vi "Add Waveform Sections.vi"(8 "error in":errorcluster, 10 "Source Waveform refs in":T1[](array[typedef]) format="%.0x", 11 "CustomDevice Ref":T1 format="%.0x") -> (0 "error out":errorcluster, 1 "Waveform Result Section refs":T1[](array[typedef]) format="%.0x", 2 "Source Waveform refs out":T1[](array[typedef]) format="%.0x", 3 "CustomDevice Ref":T1 format="%.0x")   [LabVIEW 2015, in "Waveform-Processing-Custom-Device System Explorer.lvlib"]
uses:
  Waveform-Processing-Custom-Device System Explorer.lvlib
  <vilib>/NI VeriStand/Custom Device API/Custom Device API.lvlib
  Shared/Constants.vi
  Shared/Waveform-Processing-Custom-Device Shared.lvlib
  <vilib>/NI Veristand/Custom Device API/Set Item Property (Dependent Node Pointer).vi
  NationalInstruments.VeriStand.SystemStorage
  <vilib>/NI Veristand/Custom Device API/Set Item Property (Double).vi
  <vilib>/NI Veristand/Custom Device API/Custom Device Item Ref.ctl
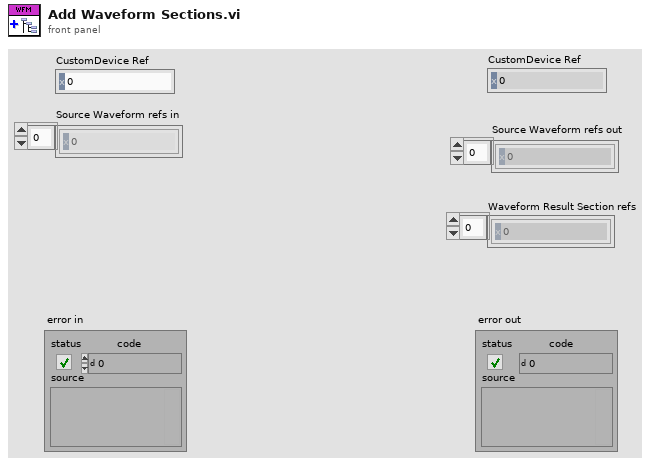
[diagram p1: front panel]
types:
  T1 = typedef "Custom Device API.lvlib/Custom Device Item Ref.ctl" = u64
  T2 = typedef "Custom Device API.lvlib/Custom Device Pointer.ctl" = refnum<k24>
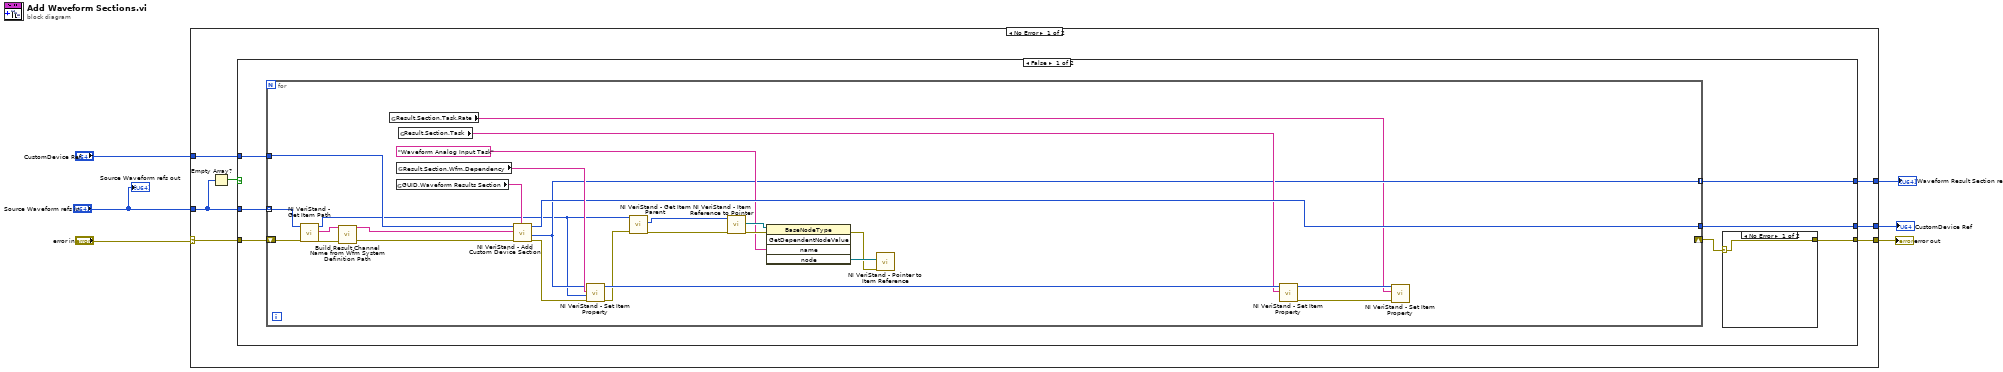
[diagram p0: block diagram]
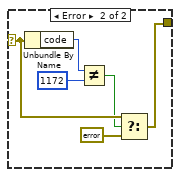
[diagram p2: hidden frame]
diagram:
  n1 = case shown="No Error" "error in" {
    selector: "error in" -> [w12 w57]
    tunnel: [w11 w57] -> w5
    tunnel: "CustomDevice Ref" -> [w13 w56]
    tunnel: [w10 w56] -> w3
    tunnel: [w8 _] -> w2
    tunnel: "Source Waveform refs in" -> [w7 _]
    frame No Error {
      n2 = Empty Array?(array=w7) -> (empty?=w9:bool)
      n3 = case shown="False" w9 {
        tunnel: w13 -> [w20 w55]
        tunnel: w12 -> [w19 w54]
        tunnel: [w16 w54] -> w11
        tunnel: [w18 w55] -> w10
        tunnel: [w15 _] -> w8
        tunnel: w7 -> [w14 _]
        frame False {
          n4 = for {
            tunnel: w20 -> [w53]
            tunnel: [w49] -> w18
            shift-right: [_] -> w17
            shift-left: w19 -> [w37]
            tunnel: [w38] -> w15 mode=indexing
            tunnel: w14 -> [w36] mode=indexing
            n5 = call <vilib>:"NI VeriStand - Get Item Path.vi"("error in (no error)"=w37, "Item Ref in"=w36) -> ("error out"=w34:errorcluster, "Path"=w33:string, "Item Ref out"=w35:T1)  [unwired: 6 in, 1 out]
            n6 = call "Build Result Channel Name from Wfm System Definition Path.vi"("error in (no error)"=w34, "Channel Path"=w33) -> ("error out"=w31:errorcluster, "delimited string"=w32:string)  [unwired: 8 in]
            n7 = global read "Constants.vi" "Result.Section.Task.Rate"() -> (w29:string)
            n8 = global read "Constants.vi" "GUID.Waveform Results Section"() -> (w52:string)
            n9 = global read "Constants.vi" "Result.Section.Wfm.Dependency"() -> (w51:string)
            n10 = global read "Constants.vi" "Result.Section.Task"() -> (w47:string)
            n11 = call <vilib>:"NI VeriStand - Add Custom Device Section.vi"("GUID (Default Section)"=w52, "error in (no error)"=w31, "Section Name"=w32, "Parent Ref in"=w53) -> ("error out"=w50:errorcluster, "Section Ptr"=w38:T1, "Parent Ref out"=w49:T1)  [unwired: 4 in, 1 out]
            n12 = call-poly <vilib>:"NI VeriStand - Set Item Property.vi"("error in (no error)"=w50, "Dependent Node Ref"=w35, "Property Name"=w51, "Item Ref in"=w38) -> ("error out"=w46:errorcluster, "Item Ref out"=w48:T1)  [unwired: 5 in, 1 out]
            n13 = call <vilib>:"NI VeriStand - Get Item Parent.vi"("error in (no error)"=w46, "Item Ref in"=w35) -> ("error out"=w45:errorcluster, "Parent Ref"=w44:T1)  [unwired: 6 in, 2 out]
            n14 = call <vilib>:"NI VeriStand - Item Reference to Pointer.vi"("error in (no error)"=w45, "Item Ref in"=w44) -> ("error out"=w42:errorcluster, "Node Pointer"=w43:T2)  [unwired: 6 in, 2 out]
            n15 = invoke class="BaseNodeType" method="GetDependentNodeValue"(reference=w43, error in=w42, "name"="Waveform Analog Input Task" ("Property Name")) -> (error out=w39:errorcluster, "node"=w40:refnum<k24>)  [unwired: 2 in, 3 out]
            n16 = call <vilib>:"NI VeriStand - Pointer to Item Reference.vi"("error in (no error)"=w39, "Node Pointer"=w40) -> ()  [unwired: 8 in, 2 out]
            n17 = call-poly <vilib>:"NI VeriStand - Set Item Property.vi"("Property Name"=w47, "Item Ref in"=w48) -> ("error out"=w28:errorcluster, "Item Ref out"=w30:T1)  [unwired: 7 in, 1 out]
            n18 = call-poly <vilib>:"NI VeriStand - Set Item Property.vi"("error in (no error)"=w28, "Property Name"=w29, "Item Ref in"=w30) -> ()  [unwired: 6 in, 3 out]
          }
          n19 = case shown="No Error" w17 {
            selector: w17 -> [w21 w25]
            tunnel: [w21 w22] -> w16
            frame No Error {
            }
            frame Error {
              n20 = Unbundle By Name(w25) -> ("code"=w27:i32)
              n21 = Not Equal?(x=w27, y=1172) -> (x != y?=w24:bool)
              n22 = Select(t=w25, s=w24, f=errorcluster {"status"=FALSE, "code"=0, "source"=""}) -> (s? t:f=w22:errorcluster)
            }
          }
        }
        frame True {
        }
      }
    }
    frame Error {
    }
  }
  "error out" <- w5
  "CustomDevice Ref" <- w3
  "Waveform Result Section refs" <- w2
  "Source Waveform refs out" <- "Source Waveform refs in"
